vi "[SubVI]Save_Config.vi"(1 "Saving File Name":string) -> (0 "Byte Stream File out":refnum<file>)   [LabVIEW 2019]
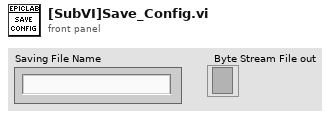
[diagram p1: front panel]
types:
  T1 = enum16{"open", "replace", "create", "open or create", "replace or create", "replace or create with confirmation"}
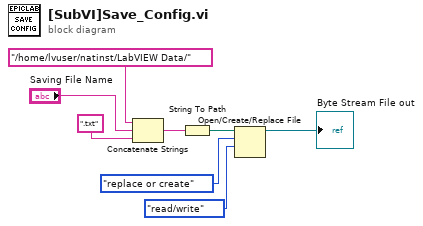
[diagram p0: block diagram]
diagram:
  n1 = Concatenate Strings("/home/lvuser/natinst/LabVIEW Data/", "Saving File Name", ".txt" ("string")) -> (w6:string)
  n2 = String To Path(string=w6) -> (path=w7:path)
  n3 = Open/Create/Replace File(file path (use dialog)=w7, operation (0:open)=T1."replace or create", access (0:read/write)=enum16{"read/write", "read-only", "write-only"}."read/write") -> (refnum out=→"Byte Stream File out":refnum<file>)  [unwired: 3 in, 2 out]
